vi "Intan_CreateBinaryFile_ExtraData.vi"(5 "DataFilePath":path=path "C:/write-read example.txt") -> (0 "Aux File Path":path, 2 "refnum out":refnum<file>)   [LabVIEW 2020]
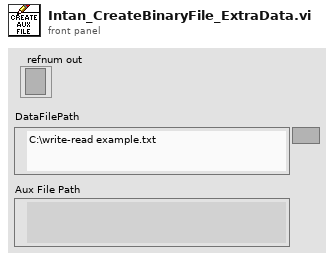
[diagram p1: front panel]
types:
  T1 = enum16{"open", "replace", "create", "open or create", "replace or create", "replace or create with confirmation"}
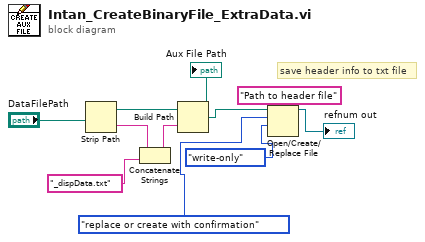
[diagram p0: block diagram]
diagram:
  (unwired) "Path to header file" ("prompt (Choose or enter file path)")
  # "save header info to txt file"
  n1 = Strip Path(path="DataFilePath") -> (stripped path=w8:path, name=w3:string)
  n2 = Concatenate Strings(w3, "_dispData.txt" ("name or relative path")) -> (w1:string)
  n3 = Build Path(base path=w8, name or relative path=w1) -> (appended path=w7:path)
  "Aux File Path" <- w7
  n4 = Open/Create/Replace File(file path (use dialog)=w7, operation (0:open)=T1."replace or create with confirmation", access (0:read/write)=enum16{"read/write", "read-only", "write-only"}."write-only") -> (refnum out=→"refnum out":refnum<file>)  [unwired: 3 in, 2 out]
